vi "CSMP-PostSendMsg.vi"(0 "State":string, 1 "Args":string, 2 "Source/target":string, 5 "Error In":errorcluster caption="error in (no error)", 6 "Session Error":errorcluster, 8 "Module Name":string, 10 "Response Arguments":string) -> (14 "State Out":string, 15 "Args Out":string, 16 "Source/target Out":string, 19 "Error":errorcluster)   [LabVIEW 2017, in "Communicable State Machine.lvlib"]
doc: "### CSMP-PostSendMsg.vi\n\n-- <b>Controls</b> --\n- <b>state</b>:\n- <b>args</b>:\n- <b>source/target</b>:\n- <b>session error</b>:\n- <b>Module Name</b>:\n- <b>Response Arguments</b>:\n\n-- <b>Indicators</b> --\n- <b>state out</b>:\n- <b>args out</b>:\n- <b>source/target out</b>:\n- <b>error</b>:"
uses:
  Communicable State Machine.lvlib
  Typedef/_Cross CSM State Response.ctl
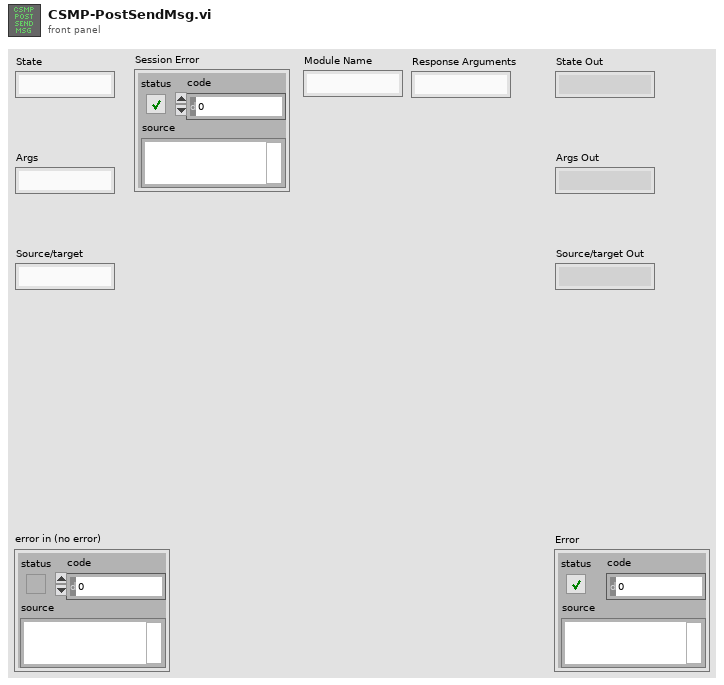
[diagram p1: front panel]
types:
  T1 = typedef "Communicable State Machine.lvlib/_Cross CSM State Response.ctl" = cluster{"error":errorcluster, "Response Data":string, "From Who":string}
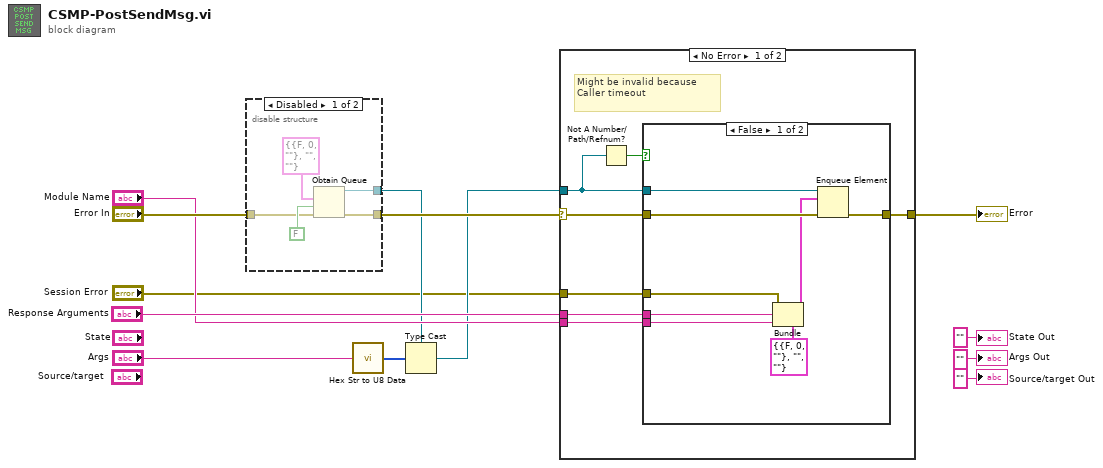
[diagram p0: block diagram]
diagram:
  n1 = disable-structure shown="Disabled" {
    disable-tunnel: [w18 _] -> w5
    disable-tunnel: [w17 _] -> w13
    disable-tunnel: "Error In" -> [w14 _]
    frame Disabled {
      n2 = Obtain Queue(element data type=T1 {"error"={"status"=FALSE, "code"=0, "source"=""}, "Response Data"="", "From Who"=""} ("Cross JKI State Machine Response"), create if not found? (T)=FALSE, error in (no error)=w14) -> (queue out=w18:refnum<queue>, error out=w17:errorcluster)  [unwired: 2 in, 1 out]
    }
    frame Enabled {
    }
  }
  n3 = call "Hex Str to U8 Data.vi"("HEX String (0-9,A-F)"="Args") -> ("U8 Data[]"=w2:u8[])
  n4 = Type Cast(type=w5, x=w2) -> (*(type *) &x=w4:refnum<queue>)
  n5 = case shown="No Error" w13 {
    selector: w13 -> [w25 w35]
    tunnel: w4 -> [w21 _]
    tunnel: [w24 w35] -> w6
    tunnel: "Module Name" -> [w23 _]
    tunnel: "Response Arguments" -> [w22 _]
    tunnel: "Session Error" -> [w19 _]
    frame No Error {
      # "Might be invalid because Caller timeout"
      n6 = Not A Number/Path/Refnum?(number/path/refnum=w21) -> (NaN/Path/Refnum?=w20:bool)
      n7 = case shown="False" w20 {
        tunnel: w25 -> [w33 w34]
        tunnel: [w32 w34] -> w24
        tunnel: w23 -> [w29 _]
        tunnel: w22 -> [w28 _]
        tunnel: w21 -> [w27 _]
        tunnel: w19 -> [w26 _]
        frame False {
          n8 = Bundle(cluster=T1 {"error"={"status"=FALSE, "code"=0, "source"=""}, "Response Data"="", "From Who"=""} ("element"), "error"=w26, "Response Data"=w28, "From Who"=w29) -> (w30:T1)
          n9 = Enqueue Element(queue=w27, element=w30, error in (no error)=w33) -> (error out=w32:errorcluster)  [unwired: 1 in, 2 out]
        }
        frame True {
        }
      }
    }
    frame Error {
    }
  }
  "Error" <- w6
  "State Out" <- "" ("Pre-State out")
  "Args Out" <- "" ("Pre-State out")
  "Source/target Out" <- "" ("Pre-Args out")
